vi "createCanFile.vi"(8 "error in":errorcluster, 11 "contentArray":string[](array[string])) -> (0 "error out":errorcluster)   [LabVIEW 2010]
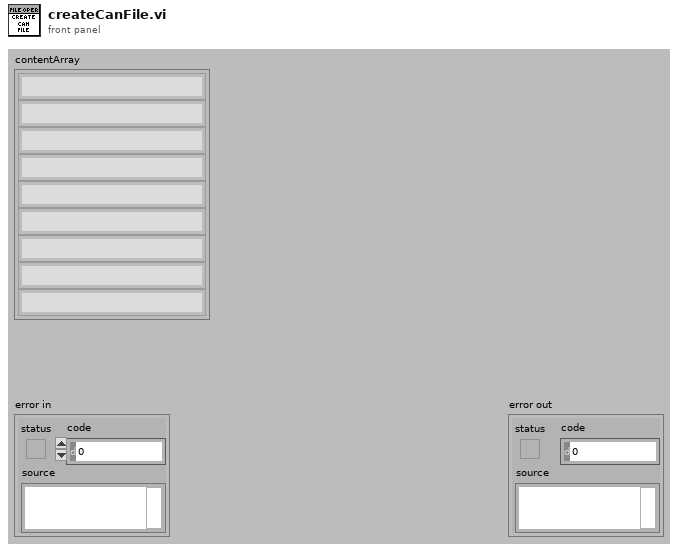
[diagram p1: front panel]
types:
  T1 = enum16{"open", "replace", "create", "open or create", "replace or create", "replace or create with confirmation"}
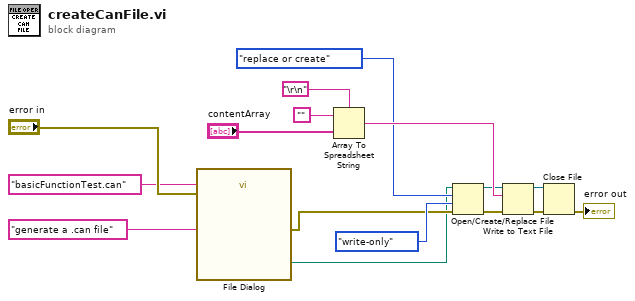
[diagram p0: block diagram]
diagram:
  n1 = call "File Dialog"("prompt"="generate a .can file", "default name"="basicFunctionTest.can" ("prompt"), "error in"="error in") -> ("selected path"=w3:path, "error out"=w5:errorcluster)  [unwired: 9 in, 2 out]
  n2 = Array To Spreadsheet String(delimiter (Tab)="\r\n", array="contentArray", 3:"") -> (spreadsheet string=w11:string)
  n3 = Open/Create/Replace File(file path (use dialog)=w3, error in=w5, operation (0:open)=T1."replace or create", access (0:read/write)=enum16{"read/write", "read-only", "write-only"}."write-only") -> (refnum out=w10:refnum<file>, error out=w12:errorcluster)  [unwired: 2 in, 1 out]
  n4 = Write to Text File(file (use dialog)=w10, text=w11, error in=w12) -> (refnum out=w14:refnum<file>, error out=w15:errorcluster)  [unwired: 1 in, 1 out]
  n5 = Close File(refnum=w14, error in=w15) -> (error out=→"error out":errorcluster)  [unwired: 1 out]
